vi "Access DB Path.vi"(9 "Password":string, 10 "ping":bool, 11 "database":string="database1.mdb") -> (2 "Connection information":string, 3 "Path out":string)   [LabVIEW 2022 SP3, in "Access Lib.lvlib"]
uses:
  Access Lib.lvlib
  <vilib>/Utility/sysdir.llb/System Directory Type.ctl
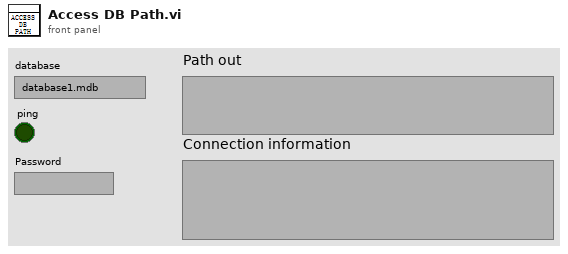
[diagram p1: front panel]
types:
  T1 = typedef "System Directory Type.ctl" = i32
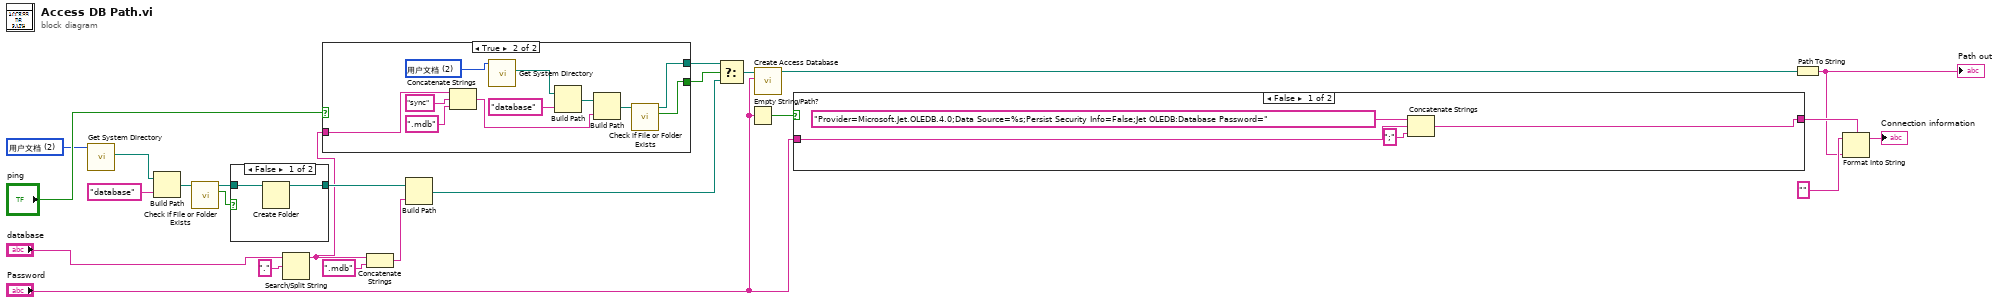
[diagram p0: block diagram]
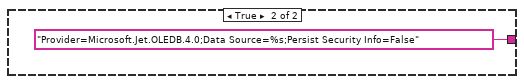
[diagram p3: hidden frame]
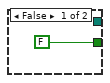
[diagram p4: hidden frame]
diagram:
  w10 = T1 2 items=["用户目录"=0, "用户桌面"=1, "用户文档"=2, "用户应用程序数据"=3, "用户设置"=4, "用户临时目录"=5, "公共文档"=6, "公共应用程序数据"=7, "公共设置"=8, "公共缓存"=13, "系统核心库"=9, "系统安装库"=10, "应用程序文件"=11, "启动盘根目录"=12] ("system directory type")
  n1 = call <vilib>:"Get System Directory.vi"("system directory type"=w10) -> ("system directory"=w9:path)  [unwired: 10 in]
  n2 = Build Path(base path=w9, name or relative path="database" ("名称或相对路径")) -> (appended path=w7:path)
  n3 = call <vilib>:"Check if File or Folder Exists.vi"("path"=w7) -> ("file or folder exists?"=w13:bool, "dup path"=w12:path)  [unwired: 8 in, 1 out]
  n4 = case shown="False" w13 {
    tunnel: w12 -> [w26 w27]
    tunnel: [w25 w27] -> w11
    frame False {
      n5 = Create Folder(path (use dialog)=w26) -> (created path=w25:path)  [unwired: 2 in, 2 out]
    }
    frame True {
    }
  }
  n6 = Search/Split String(string="database", search string/char (-)="." ("搜索字符串/字符(-)")) -> (substring before match=w1:string)  [unwired: 1 in, 2 out]
  n7 = case shown="True" "ping" {
    tunnel: [FALSE ("file or folder exists?") w34] -> w6
    tunnel: [_ w33] -> w5
    tunnel: w1 -> [_ w29]
    frame False {
    }
    frame True {
      w39 = T1 2 items=["用户目录"=0, "用户桌面"=1, "用户文档"=2, "用户应用程序数据"=3, "用户设置"=4, "用户临时目录"=5, "公共文档"=6, "公共应用程序数据"=7, "公共设置"=8, "公共缓存"=13, "系统核心库"=9, "系统安装库"=10, "应用程序文件"=11, "启动盘根目录"=12] ("system directory type")
      n8 = Concatenate Strings(w29, "sync" ("字符串"), ".mdb" ("字符串")) -> (w30:string)
      n9 = call <vilib>:"Get System Directory.vi"("system directory type"=w39) -> ("system directory"=w38:path)  [unwired: 10 in]
      n10 = Build Path(base path=w38, name or relative path="database" ("名称或相对路径")) -> (appended path=w36:path)
      n11 = Build Path(base path=w36, name or relative path=w30) -> (appended path=w35:path)
      n12 = call <vilib>:"Check if File or Folder Exists.vi"("path"=w35) -> ("file or folder exists?"=w34:bool, "dup path"=w33:path)  [unwired: 8 in, 1 out]
    }
  }
  n13 = Concatenate Strings(w1, ".mdb" ("字符串")) -> (w2:string)
  n14 = Build Path(base path=w11, name or relative path=w2) -> (appended path=w4:path)
  n15 = Select(t=w5, s=w6, f=w4) -> (s? t:f=w3:path)
  n16 = Empty String/Path?(string/path="Password") -> (empty?=w22:bool)
  n17 = call "Create Access Database.vi"("Password"="Password", "路径"=w3) -> ("路径 out"=w23:path)  [unwired: 8 in, 1 out]
  n18 = case shown="False" w22 {
    tunnel: [w40 "Provider=Microsoft.Jet.OLEDB.4.0;Data Source=%s;Persist Security Info=False" ("格式字符串")] -> w20
    tunnel: "Password" -> [w43 _]
    frame False {
      n19 = Concatenate Strings("Provider=Microsoft.Jet.OLEDB.4.0;Data Source=%s;Persist Security Info=False;Jet OLEDB:Database Password=" ("格式字符串"), w43, ";" ("字符串")) -> (w40:string)
    }
    frame True {
    }
  }
  n20 = Path To String(path=w23) -> (string=w18:string)
  "Path out" <- w18
  n21 = Format Into String(format string=w20, initial string="" ("初始字符串"), w18) -> (resulting string=→"Connection information":string)  [unwired: 1 in, 1 out]
